vi "cno_update Hessian.vi"(4 "SX":dbl[](array[numeric]), 5 "G":dbl[](array[numeric]), 6 "P":dbl[](array[numeric]), 7 "YG":dbl[](array[numeric]), 8 "error in (no error)":errorcluster, 11 "H":dbl[][](array[numeric])) -> (0 "error out":errorcluster, 3 "H":dbl[][](array[numeric]))   [LabVIEW 2018, in "NI_Gmath.lvlib"]
uses:
  NI_Gmath.lvlib
  Real Dot Product.vi
  A x Vector.vi
  Real Outer Product.vi
  Array To Matrix - RA2.vi
  Matrix To Array - RM.vi
  <vilib>/Analysis/NI_AALBase.lvlib
  NI_Matrix.lvlib
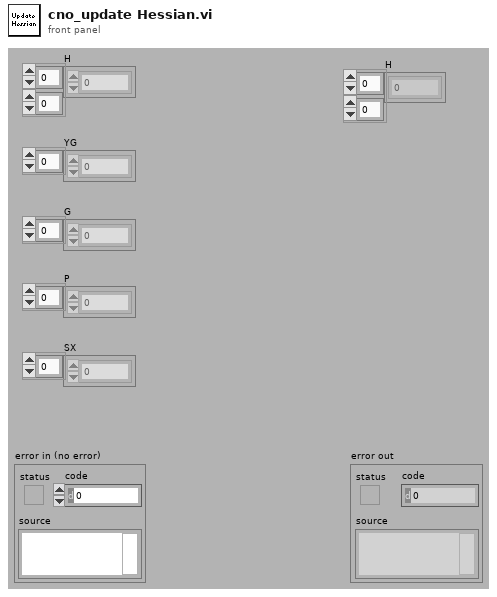
[diagram p1: front panel]
types:
  T1 = typedef "NI_Matrix.lvlib/RealMatrix.ctl" = dbl[][]
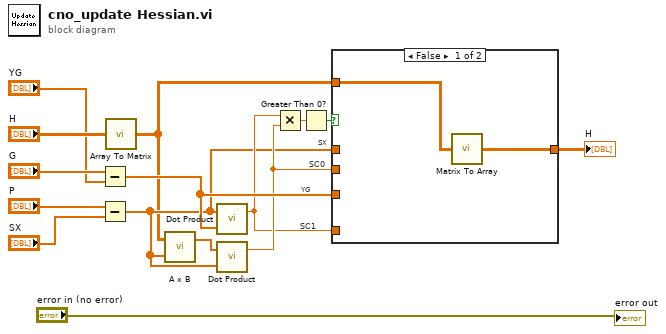
[diagram p0: block diagram]
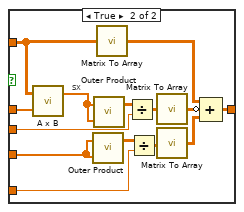
[diagram p2: hidden frame]
diagram:
  # "YG"
  # "SC0"
  # "SC1"
  # "SX"
  n1 = Subtract(x="G", y="YG") -> (x-y=w14:dbl[])
  n2 = Subtract(x="P", y="SX") -> (x-y=w11:dbl[])
  n3 = call-poly "Array To Matrix.vi"("Real 2D Array"="H") -> ("Real Matrix"=w1:T1)
  n4 = call-poly "A x B.vi"("Vector"=w11, "A"=w1) -> ("A x Vector"=w6:dbl[])  [unwired: 1 out]
  n5 = call-poly "Dot Product.vi"("Y Vector"=w14, "X Vector"=w11) -> ("X * Y"=w12:dbl)  [unwired: 1 out]
  n6 = call-poly "Dot Product.vi"("Y Vector"=w11, "X Vector"=w6) -> ("X * Y"=w13:dbl)  [unwired: 1 out]
  n7 = Multiply(x=w12, y=w13) -> (x*y=w8:dbl)
  n8 = Greater Than 0?(x=w8) -> (x > 0?=w9:bool)
  n9 = case shown="False" w9 {
    tunnel: w11 -> [_ w31]
    tunnel: w1 -> [w17 w25]
    tunnel: w12 -> [_ w26]
    tunnel: w13 -> [_ w29]
    tunnel: w14 -> [_ w28]
    tunnel: [w16 w22] -> w15
    frame False {
      n10 = call-poly "Matrix To Array.vi"("Real Matrix"=w17) -> ("Real 2D Array"=w16:dbl[][])
    }
    frame True {
      # "SX"
      n11 = call-poly "A x B.vi"("Vector"=w31, "A"=w25) -> ("A x Vector"=w21:dbl[])  [unwired: 1 out]
      n12 = call-poly "Outer Product.vi"("Y Vector"=w28, "X Vector"=w28) -> ("Outer Product"=w27:T1)  [unwired: 1 out]
      n13 = call-poly "Outer Product.vi"("Y Vector"=w21, "X Vector"=w21) -> ("Outer Product"=w30:T1)  [unwired: 1 out]
      n14 = call-poly "Matrix To Array.vi"("Real Matrix"=w25) -> ("Real 2D Array"=w18:dbl[][])
      n15 = Divide(x=w30, y=w29) -> (x/y=w24:T1)
      n16 = Divide(x=w27, y=w26) -> (x/y=w23:T1)
      n17 = call-poly "Matrix To Array.vi"("Real Matrix"=w24) -> ("Real 2D Array"=w20:dbl[][])
      n18 = call-poly "Matrix To Array.vi"("Real Matrix"=w23) -> ("Real 2D Array"=w19:dbl[][])
      n19 = Compound Arithmetic op=ADD(w18, invert w20, w19) -> (w22:dbl[][])
    }
  }
  "H" <- w15
  "error out" <- "error in (no error)"
